vi "Construct Event Message Callback.vi"() -> (0 "error out":errorcluster, 2 "Message Received Callback":refnum<user-event>, 3 "EventMessageRxCallback out":refnum<class "EventMessageRxCallback.lvclass">)   [LabVIEW 2019, in "EventMessageRxCallback.lvclass"]
uses:
  <vilib>/gpm_packages/@cs/Network-interface/Examples/EventMessageRxCallback/EventMessageRxCallback.lvclass
  <vilib>/gpm_packages/@cs/Network-interface/Examples/EventMessageRxCallback/Message Information Type.ctl
  <vilib>/gpm_packages/@cs/Network-interface/Examples/EventMessageRxCallback/EventMessageRxCallback.lvclass/EventMessageRxCallback.ctl
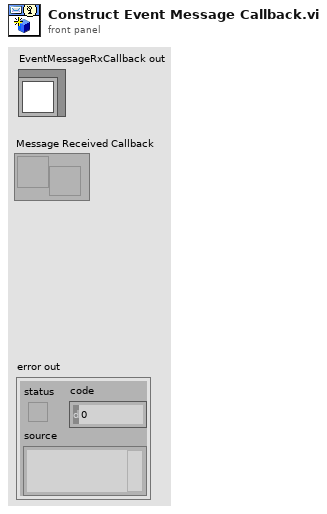
[diagram p1: front panel]
types:
  T1 = typedef "EventMessageRxCallback.lvclass/Message Information Type.ctl" = cluster{"Connection ID":string, "Message":string, "Data":variant}
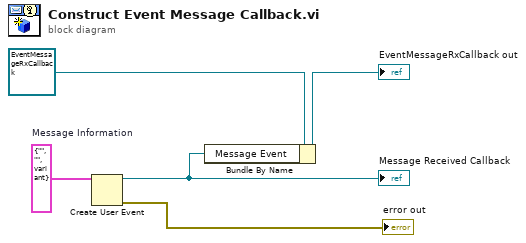
[diagram p0: block diagram]
diagram:
  w4 = T1 {"Connection ID"="", "Message"="", "Data"=variant}  # Message Information
  n1 = Create User Event(user event datatype=w4) -> (user event=w2:refnum<user-event>, error out=→"error out":errorcluster)  [unwired: 1 in]
  "Message Received Callback" <- w2
  n2 = Bundle By Name(cluster=refnum<class "EventMessageRxCallback.lvclass"> refnum ("EventMessageRxCallback in"), "Message Event"=w2) -> (→"EventMessageRxCallback out":refnum<class "EventMessageRxCallback.lvclass">)
